vi "ConfigGLOB.vi"() -> ()   [LabVIEW 2015, in "Tool Cfg.lvlib"]
uses:
  Tool Cfg.lvlib
  _Configuration Cluster_v3--typedef.ctl
  _Tool Block Cluster_v3--typedef.ctl
  _Motor Block Cluster_v2--typedef.ctl
  _Verification Blk Cluster--typedef.ctl
  _ProbeConfigParams Cluster--typedef.ctl
  _Sensor Block Cluster--typedef.ctl
  _SensorConfigParams Cluster--typedef.ctl
  _Tool Operation Config Cluster--typedef.ctl
panel:
  in  "Firware Version":string
  in  "Product Name":string="QC-X Thread Profiler"
  in  "Tool Operation Config":T1={"Use Tool Cfg"=TRUE, "Use Tool Cal"=TRUE, "Fake Data?"=FALSE, "Mode"=-2, "Array Subset Length"=512, "nArrays to Read"=2, "Full Array Read Length"=512, "nSubarrays/Sensor"=1}
  in  "Config Cluster Version":string="3"
  in  "Tool Config Cluster":T2={"Tool Type"=12, "Tool SN"=103, "Tool Block"={"Encoder Size"=1, "Encoder Scale"=635000, "Encoder Offset"=20000, "MaxEncoder"=3175000, "MinEncoder"=0, "Start Delay"=0.015, "Tool Face Ref"=0.0}, "Motor Block"={"MinMotor Speed"=120, "MaxMotor Speed"=3500, "Homing Speed"=350, "Jog Speed"=560, "Inspect Speed"=480, "VBlk Speed"=452, "CleaningPos"=635000, "Safe Zone"=635000, "Has Motor"=TRUE, "Use Home Index"=TRUE}, "Verification Block"={"Angle"=90.0, "FlankLength1"=0.28, "FlankLength2"=0.28, "Location"=0.45, "Serial Number"=101}, "Probe Block"={"nProbes"=2, "Probe Param Array"=[{"Name"="Lead", "Laser Init Pwr"=2110, "Laser Gain"=8, "Integ Count"=300, "Meas. Range"=0.3, "Angle"=-20.66978, "Probe Offset"=0.0, "Sensor Block"={"nSensors"=1, "SensorCfgParams Array"=[{"Total Pixels"=512, "Positive  Peaks"=TRUE, "CalibrCoefArray"=[-0.0293110138012284, 0.18436244198429, 0.0375363053051945, 0.20167602015109, -0.19043592344047, 0.14097372183574], "Start Idx"=0, "End Idx"=0}]}}, {"Name"="Lag", "Laser Init Pwr"=2110, "Laser Gain"=8, "Integ Count"=300, "Meas. Range"=0.3, "Angle"=19.16363, "Probe Offset"=-0.3029, "Sensor Block"={"nSensors"=1, "SensorCfgParams Array"=[{"Total Pixels"=512, "Positive  Peaks"=TRUE, "CalibrCoefArray"=[-0.0277273717873249, 0.18323721389216, 0.0298372208825187, 0.21864598966908, -0.20014016741566, 0.14218856057391], "Start Idx"=0, "End Idx"=0}]}}]}} {"Probe Block"."Probe Param Array"."Sensor Block"."SensorCfgParams Array"."CalibrCoefArray" format="%#.12g"}
  # "The Tool Config Cluster comes from the\nQCX Tool Cfg.xml file on the RT file system."
  # "Note: this is not use.\nFirmware version is set in RT MAIN.vi"
  # "The Tool Operation Config\ncomes from the PC App."
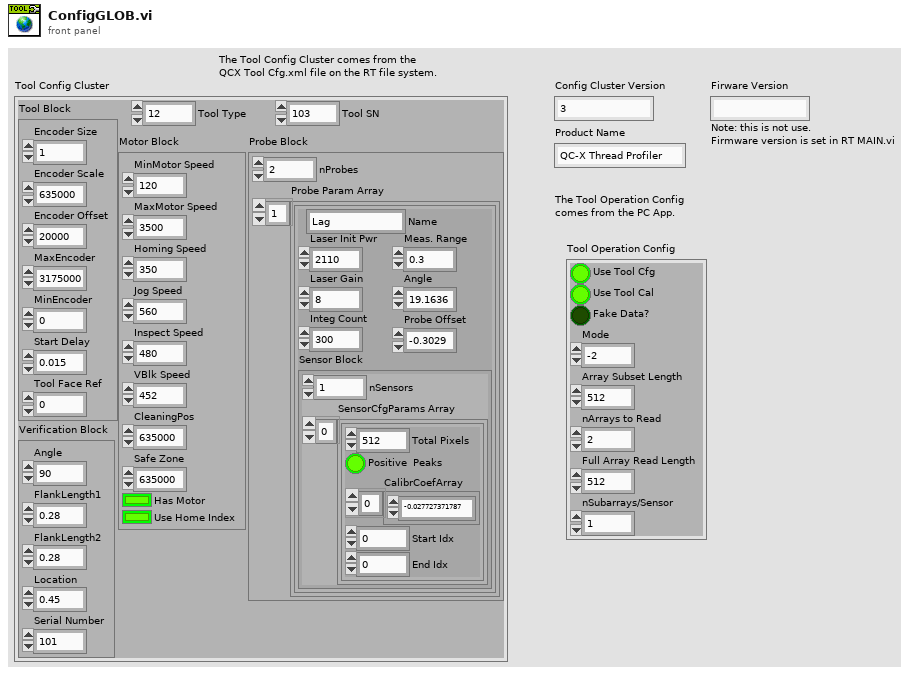
[diagram p1: front panel]
types:
  T1 = typedef "Tool Cfg.lvlib/_Tool Operation Config Cluster--typedef.ctl" = cluster{"Use Tool Cfg":bool, "Use Tool Cal":bool, "Fake Data?":bool, "Mode":i16, "Array Subset Length":i16, "nArrays to Read":i16, "Full Array Read Length":i16, "nSubarrays/Sensor":i16}
  T2 = typedef "Tool Cfg.lvlib/_Configuration Cluster_v3--typedef.ctl" = cluster{"Tool Type":u16, "Tool SN":u16, "Tool Block":T3, "Motor Block":T4, "Verification Block":T5, "Probe Block":cluster{"nProbes":u16, "Probe Param Array":T6[]}}
  T3 = typedef "Tool Cfg.lvlib/_Tool Block Cluster_v3--typedef.ctl" = cluster{"Encoder Size":u16, "Encoder Scale":u32, "Encoder Offset":i32, "MaxEncoder":i32, "MinEncoder":i32, "Start Delay":sgl, "Tool Face Ref":sgl}
  T4 = typedef "Tool Cfg.lvlib/_Motor Block Cluster_v2--typedef.ctl" = cluster{"MinMotor Speed":u16, "MaxMotor Speed":u16, "Homing Speed":u16, "Jog Speed":u16, "Inspect Speed":u16, "VBlk Speed":u16, "CleaningPos":i32, "Safe Zone":i32, "Has Motor":bool, "Use Home Index":bool}
  T5 = typedef "Tool Cfg.lvlib/_Verification Blk Cluster--typedef.ctl" = cluster{"Angle":sgl, "FlankLength1":sgl, "FlankLength2":sgl, "Location":sgl, "Serial Number":u16}
  T6 = typedef "Tool Cfg.lvlib/_ProbeConfigParams Cluster--typedef.ctl" = cluster{"Name":string, "Laser Init Pwr":u16, "Laser Gain":u8, "Integ Count":u16, "Meas. Range":sgl, "Angle":sgl, "Probe Offset":sgl, "Sensor Block":T7}
  T7 = typedef "Tool Cfg.lvlib/_Sensor Block Cluster--typedef.ctl" = cluster{"nSensors":u16, "SensorCfgParams Array":T8[]}
  T8 = typedef "Tool Cfg.lvlib/_SensorConfigParams Cluster--typedef.ctl" = cluster{"Total Pixels":u16, "Positive  Peaks":bool, "CalibrCoefArray":dbl[], "Start Idx":u16, "End Idx":u16}
diagram:
